vi "alignment_sub.vi"() -> ()   [LabVIEW 2011]
uses:
  global_vars.vi
panel:
  in  "u16_choose_cam":u16(ring)=1 items=[" HP Cam", "PixelLink Cam"]
  in  "dbl_shutter_value":dbl(slide)=0.036604516208171844 caption="Camera Shutter \n(PixelLink only)" min=0.001 max=1.0 scale=0.0..1.0
  out "Camera Stream":T1(plugin-control)
  in  "b_stream_window":bool caption="camera stream \nin extra window"
  in  "b_overlay_stream":bool caption="camera \noverlay"
  in  "i32_stream_OL_center_radius":dbl caption="center radius"
  in  "i32_stream_OL_#rings":i32=30 caption="#rings"
  in  "stream_OL_color":u32(colorbox)=16448250 caption="overlay color"
  in  "df_intial phase shift":dbl caption="intial phase shift"
  in  "i32_width":i32=500 caption="Width (Px)"
  in  "i32_height":i32=500 caption="Height (Px)"
  in  "df_#fringes":dbl=4.0 caption="#fringes"
  in  "save image of\ncamera stream":bool
  in  "File Path":path=path "X:/Cloud Drives/Dropbox/Europhotonics/FringeMan/Image Storage"
  in  "b_flip_direction":bool
  in  "i32_fringe_OL_#rings":i32=20 caption="#rings"
  in  "i32_fringe_OL_center_radius":dbl caption="center radius"
  in  "overlay color":u32(colorbox)=16448250
  in  "b_align":bool caption="fringe \noverlay"
  in  "b_preview fringes":bool=TRUE caption="preview \nfringes"
  in  "b_fit_to_screen":bool=TRUE
  in  "b_to_2nd_screen":bool=TRUE
  in  "b_close":bool
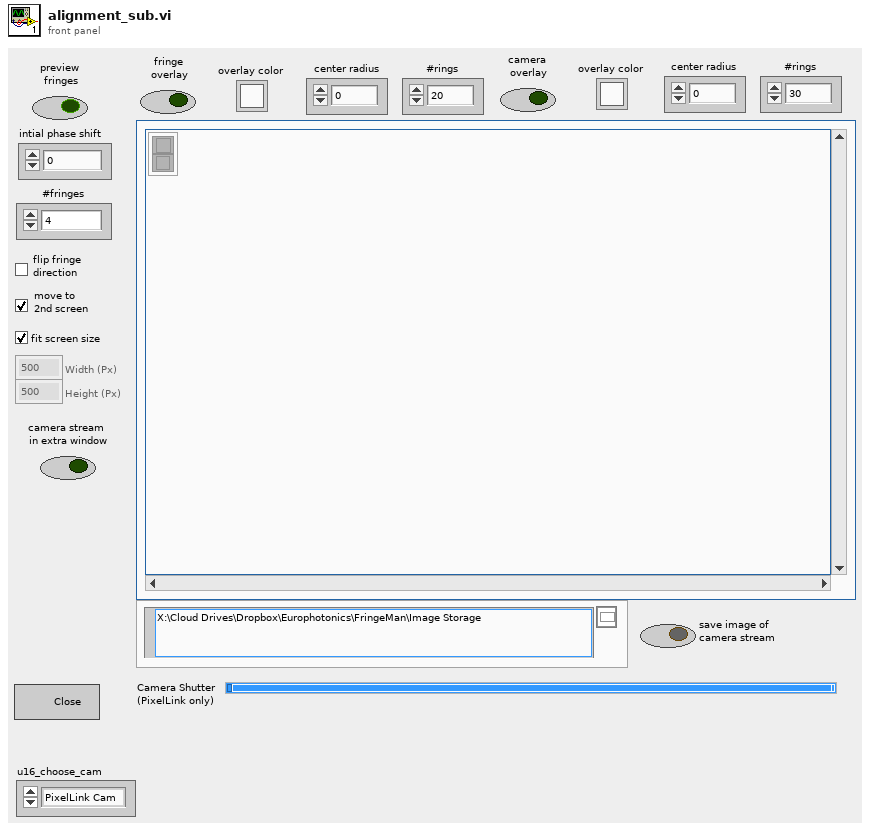
[diagram p1: front panel]
types:
  T1 = typedef "IMAQ Image.ctl" = refnum<image>
  T2 = enum8{"Enabled", "Disabled", "Disabled and Grayed Out"}
  T3 = cluster{"Numeric Control":i16, "Numeric Control":i16}
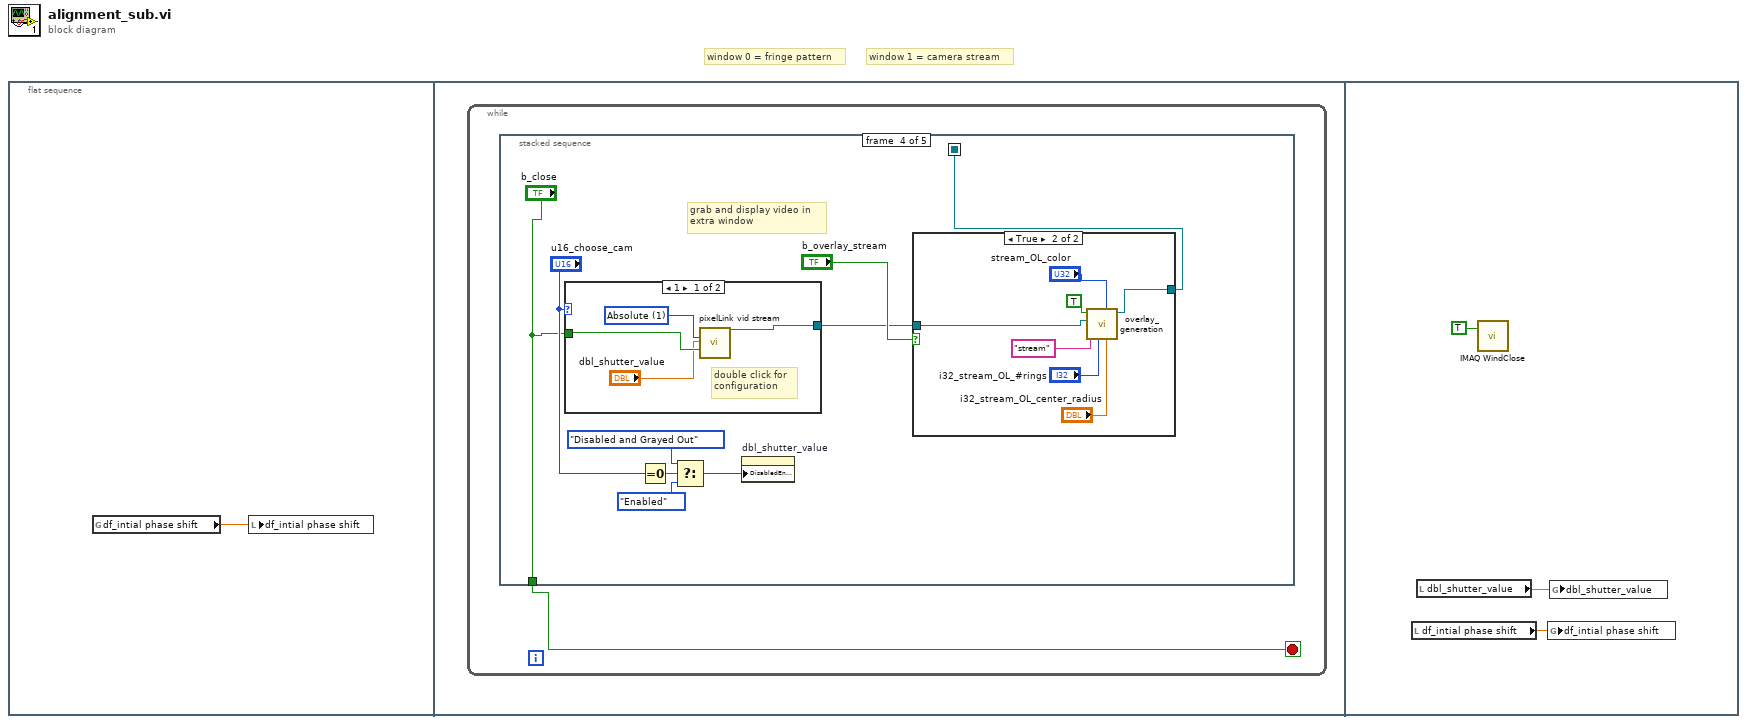
[diagram p0: block diagram]
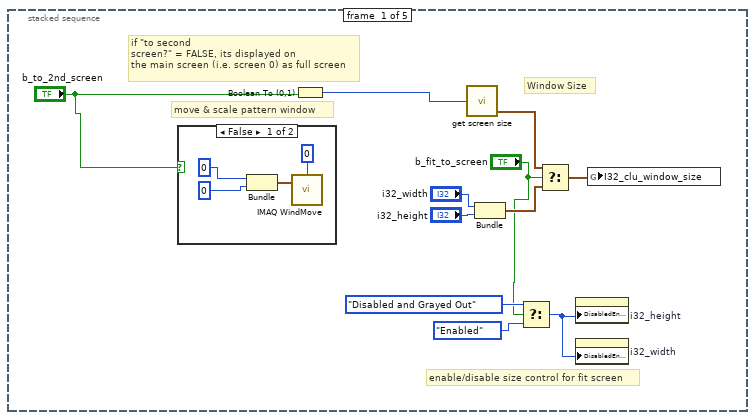
[diagram p2: hidden frame]
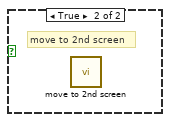
[diagram p3: hidden frame]
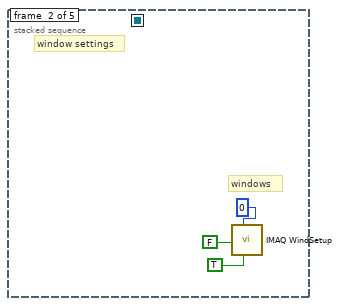
[diagram p4: hidden frame]
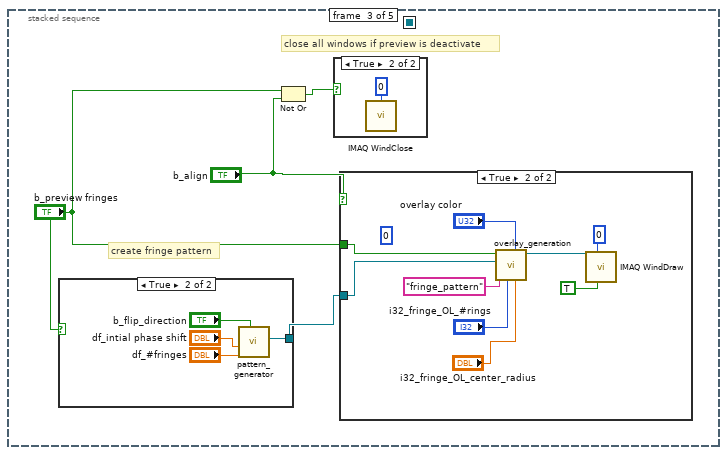
[diagram p5: hidden frame]
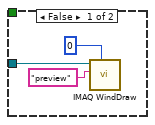
[diagram p7: hidden frame]
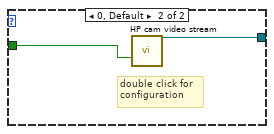
[diagram p9: hidden frame]
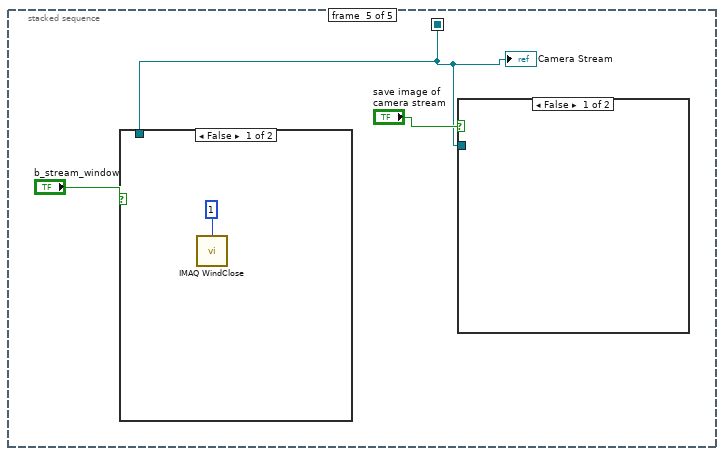
[diagram p11: hidden frame]
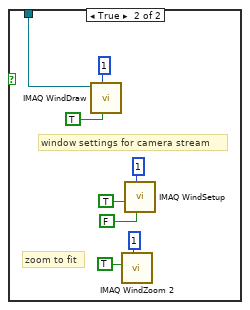
[diagram p12: hidden frame]
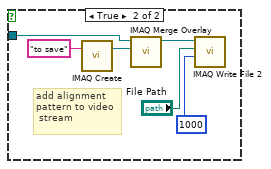
[diagram p13: hidden frame]
diagram:
  # "window 1 = camera stream"
  # "window 0 = fringe pattern"
  n1 = flat-sequence {
    frame #0 {
      n2 = global read "global_vars.vi" "df_intial phase shift"() -> (w1:dbl)
      n3 = local write "df_intial phase shift"(w1) -> ()
    }
    frame #1 {
      n4 = while {
        stop <- w2 stop-if-true
        n5 = stacked-sequence {
          seq-local: [_ _ _ w50 _] -> [_ _ _ _ w65]
          tunnel: [_ _ _ "b_close" _] -> w2
          frame #0 {
            # "enable/disable size control for fit screen"
            # "if \"to second \nscreen?\" = FALSE, its displayed on \nthe main screen (i.e. screen 0) as full screen"
            # "Window Size"
            # "move & scale pattern window"
            n6 = case shown="False" "b_to_2nd_screen" {
              frame False {
                n7 = Bundle(0, 0) -> (w17:cluster{i32, i32})  [unwired: 1 in]
                n8 = call "IMAQ WindMove"("Window Number (0...15)"=0, "Coordinates (screen)"=w17) -> ()  [unwired: 3 in, 2 out]
              }
              frame True {
                # "move to 2nd screen"
                n9 = call "move to 2nd screen.vi"() -> ()  [unwired: 12 in]
              }
            }
            n10 = Boolean To (0,1)(Boolean="b_to_2nd_screen") -> (0, 1=w13:i16)
            n11 = call "get screen size.vi"("screen"=w13) -> ("wind size (width/height)"=w12:T3)  [unwired: 2 in, 2 out]
            n12 = Bundle("i32_width"="i32_width", "i32_height"="i32_height") -> (w10:cluster{"i32_width":i32, "i32_height":i32})  [unwired: 1 in]
            n13 = Select(t=T2."Disabled and Grayed Out" ("Disabled"), s="b_fit_to_screen", f=T2."Enabled" ("Disabled")) -> (s? t:f=w3:T2)
            n14 = Select(t=w12, s="b_fit_to_screen", f=w10) -> (s? t:f=w11:cluster{"i32_width":i32, "i32_height":i32})
            n15 = property on="i32_height" class="DigNum (strict)"("DisabledEnum"=w3) -> ()  [unwired: 2 in, 2 out]
            n16 = property on="i32_width" class="DigNum (strict)"("DisabledEnum"=w3) -> ()  [unwired: 2 in, 2 out]
            n17 = global write "global_vars.vi" "I32_clu_window_size"(w11) -> ()
          }
          frame #1 {
            # "window settings"
            # "windows"
            n18 = call "IMAQ WindSetup"("Window is floating? (No)"=TRUE, "Window Number (0...15)"=0, "Window has title bar? (Yes)"=FALSE) -> ()  [unwired: 8 in, 1 out]
          }
          frame #2 {
            # "close all windows if preview is deactivate"
            # "create fringe pattern"
            n19 = case shown="True" "b_preview fringes" {
              tunnel: [_ w41] -> w21
              frame False {
              }
              frame True {
                n20 = call "pattern_generator.vi"("flip direction"="b_flip_direction", "fringe number"="df_#fringes", "phase"="df_intial phase shift") -> ("fringe pattern"=w41:T1)  [unwired: 7 in, 1 out]
              }
            }
            n21 = Not Or(1:"b_align", 2:"b_preview fringes") -> (0:w22:bool)
            n22 = case shown="True" w22 {
              frame False {
              }
              frame True {
                n23 = call "IMAQ WindClose"("Window Number (0...15)"=0) -> ()  [unwired: 5 in, 1 out]
              }
            }
            n24 = case shown="True" "b_align" {
              tunnel: w21 -> [w27 w37]
              tunnel: "b_preview fringes" -> [_ w36]
              frame False {
                n25 = call "IMAQ WindDraw"("Window Number (0...15)"=0, "Title"="preview", "Image"=w27) -> ()  [unwired: 7 in, 2 out]
              }
              frame True {
                (unwired) 0 ("Window Number (0...15)")
                n26 = call "overlay_generation.vi"("center radius"="i32_fringe_OL_center_radius", "Color"="overlay color", "number of rings"="i32_fringe_OL_#rings", "Title"="fringe_pattern", "Image Src"=w37, "fringe preview on"=w36) -> ("stream_overlay_out"=w29:T1)  [unwired: 5 in]
                n27 = call "IMAQ WindDraw"("Resize to Image Size? (Y)"=TRUE, "Window Number (0...15)"=0, "Image"=w29) -> ()  [unwired: 7 in, 2 out]
              }
            }
          }
          frame #3 {
            # "grab and display video in \nextra window"
            n28 = case shown="1" "u16_choose_cam" {
              tunnel: [w54 w56] -> w42
              tunnel: "b_close" -> [w53 w55]
              frame 1 {
                w52 = u32 1 items=["Absolute"=1, "Auto"=3, "Relative"=0, "One Push"=4, "Ignored"=5] ("Shutter::Mode")
                # "double click for\nconfiguration"
                n29 = call "pixelLink vid stream"("Shutter::Mode"=w52, "Shutter::Value"="dbl_shutter_value", "Stop (F)"=w53) -> ("Image Out"=w54:T1)  [unwired: 20 in, 4 out]
              }
              frame 0, Default {
                # "double click for\nconfiguration"
                n30 = call "HP cam video stream"("Stop (F)"=w55) -> ("Image Out"=w56:T1)  [unwired: 22 in, 4 out]
              }
            }
            n31 = Equal To 0?(x="u16_choose_cam") -> (x = 0?=w44:bool)
            n32 = Select(t=T2."Disabled and Grayed Out" ("Disabled"), s=w44, f=T2."Enabled" ("Disabled")) -> (s? t:f=w47:T2)
            n33 = property on="dbl_shutter_value" class="Slide (strict)"("DisabledEnum"=w47) -> ()  [unwired: 2 in, 2 out]
            n34 = case shown="True" "b_overlay_stream" {
              tunnel: w42 -> [w57 w59]
              tunnel: [w57 w58] -> w50
              frame False {
              }
              frame True {
                n35 = call "overlay_generation.vi"("center radius"="i32_stream_OL_center_radius", "Color"="stream_OL_color", "number of rings"="i32_stream_OL_#rings", "Title"="stream", "Image Src"=w59, "fringe preview on"=TRUE) -> ("stream_overlay_out"=w58:T1)  [unwired: 5 in]
              }
            }
          }
          frame #4 {
            n36 = case shown="False" "b_stream_window" {
              tunnel: w65 -> [_ w74]
              frame False {
                n37 = call "IMAQ WindClose"("Window Number (0...15)"=1) -> ()  [unwired: 5 in, 1 out]
              }
              frame True {
                # "zoom to fit"
                # "window settings for camera stream"
                n38 = call "IMAQ WindDraw"("Resize to Image Size? (Y)"=TRUE, "Window Number (0...15)"=1, "Image"=w74) -> ()  [unwired: 7 in, 2 out]
                n39 = call "IMAQ WindZoom 2"("Window Number (0...15)"=1, "Zoom to Fit? (False)"=TRUE) -> ()  [unwired: 6 in, 4 out]
                n40 = call "IMAQ WindSetup"("Window is floating? (No)"=FALSE ("b_floating"), "Window Number (0...15)"=1, "Window has title bar? (Yes)"=TRUE ("b_title_bar")) -> ()  [unwired: 8 in, 1 out]
              }
            }
            n41 = case shown="False" "save image of\ncamera stream" {
              tunnel: w65 -> [_ w78]
              frame False {
              }
              frame True {
                # "add alignment\npattern to video\n stream"
                n42 = call "IMAQ Create"("Image Name"="to save") -> ("New Image"=w80:T1)  [unwired: 3 in, 2 out]
                n43 = call "IMAQ Merge Overlay"("Image Dst"=w80, "Image Src"=w78) -> ("Image Dst Out"=w77:T1)  [unwired: 8 in, 1 out]
                n44 = call-poly "IMAQ Write File 2"("Image Quality"=u32 1000, "File Path"="File Path", "Image"=w77) -> ()  [unwired: 7 in, 2 out]
              }
            }
            "Camera Stream" <- w65
          }
        }
      }
    }
    frame #2 {
      n45 = local read "df_intial phase shift"() -> (w85:dbl)
      n46 = local read "dbl_shutter_value"() -> (w83:dbl)
      n47 = call "IMAQ WindClose"("Close All Windows (False)"=TRUE) -> ()  [unwired: 5 in, 1 out]
      n48 = global write "global_vars.vi" "df_intial phase shift"(w85) -> ()
      n49 = global write "global_vars.vi" "dbl_shutter_value"(w83) -> ()
    }
  }
